vi "main(Test DQMH modules).vi"() -> ()   [LabVIEW 2018, in "Application.lvlib"] (continued)
        n4329 = Or(x=w9739, y=w9737) -> (x .or. y?=w9738:bool)
        n4330 = case shown="False" w9738 {
          tunnel: [w9767 _] -> w9749
          tunnel: w9746 -> [w9766 _]
          frame False {
            w9755 = T9 {"command"="", "data"=variant} ("element")
            w9754 = "MEAS.mux6_1"
            n4331 = To Variant(anything=T2."mux6_1_channel3_3" ("mux6_1(3wires)_encode")) -> (Variant=w9764:variant)
            n4332 = To Variant(anything=T2."mux6_1_channel3_2" ("mux6_1(3wires)_encode")) -> (Variant=w9762:variant)
            n4333 = Bundle By Name(cluster=w9755, "command"=w9754, "data"=w9762) -> (w9761:T9)
            n4334 = Bundle By Name(cluster=w9755, "command"=w9754, "data"=w9764) -> (w9760:T9)
            n4335 = Bundle By Name(cluster=w9755, "command"="MEAS.DMM dual read") -> (w9758:T9)
            n4336 = Build Array(w9761, w9760, w9758) -> (w9756:T9[])
            n4337 = Reverse 1D Array(array=w9756) -> (reversed array=w9757:T9[])
            n4338 = for {
              tunnel: [w9773] -> w9767 mode=indexing
              tunnel: w9766 -> [w9772]
              tunnel: w9757 -> [w9771] mode=indexing
              n4339 = Unbundle By Name(w9771) -> ("command"=w9770:string, "data"=w9769:variant)
              n4340 = call "App enquece.vi"("Priority Enquece"=TRUE, "command data"=w9769, "command"=w9770, "queue in"=w9772) -> ("error out"=w9773:errorcluster)  [unwired: 6 in, 1 out]
            }
          }
          frame True {
          }
        }
        n4341 = Merge Errors(w9747, w9749) -> (w9748:errorcluster)
      }
      frame "Test DRV 58" {
        w9782 = 58  # DUT index(1-60)
        n4342 = disable-structure shown="LOGGING==TRUE" {
          disable-tunnel: w9783 -> [w9816 _]
          frame condition #0 (active) {
            n4343 = Empty String/Path?(string/path=w9816) -> (empty?=w9818:bool)
            n4344 = Select(t="Quece timeout", s=w9818, f=w9816) -> (s? t:f=w9815:string)
            n4345 = call "string log (SubVI).vi"("state Name"=w9815) -> ()  [unwired: 9 in, 2 out]
          }
          frame condition #1 {
          }
        }
        n4346 = call "progress string(SubVI).vi"("String 3"=w9783, "String in"=w9784) -> ("String out"=w9785:string)  [unwired: 9 in]
        n4347 = call "FGV DRV stand.vi"() -> ("Sub-Test.DCV"=w9781:bool)  [unwired: 10 in, 1 out]
        n4348 = call "FGV Driver Data.vi"("DUT index(1-60)"=w9782) -> ("DUT SC"=w9780:bool)  [unwired: 7 in, 3 out]
        n4349 = Not(x=w9781) -> (.not. x?=w9778:bool)
        n4350 = Or(x=w9780, y=w9778) -> (x .or. y?=w9779:bool)
        n4351 = case shown="False" w9779 {
          tunnel: [w9808 _] -> w9790
          tunnel: w9787 -> [w9807 _]
          frame False {
            w9796 = T9 {"command"="", "data"=variant} ("element")
            w9795 = "MEAS.mux6_1"
            n4352 = To Variant(anything=T2."mux6_1_channel4_3" ("mux6_1(3wires)_encode")) -> (Variant=w9805:variant)
            n4353 = To Variant(anything=T2."mux6_1_channel4_2" ("mux6_1(3wires)_encode")) -> (Variant=w9803:variant)
            n4354 = Bundle By Name(cluster=w9796, "command"=w9795, "data"=w9803) -> (w9802:T9)
            n4355 = Bundle By Name(cluster=w9796, "command"=w9795, "data"=w9805) -> (w9801:T9)
            n4356 = Bundle By Name(cluster=w9796, "command"="MEAS.DMM dual read") -> (w9799:T9)
            n4357 = Build Array(w9802, w9801, w9799) -> (w9797:T9[])
            n4358 = Reverse 1D Array(array=w9797) -> (reversed array=w9798:T9[])
            n4359 = for {
              tunnel: [w9814] -> w9808 mode=indexing
              tunnel: w9807 -> [w9813]
              tunnel: w9798 -> [w9812] mode=indexing
              n4360 = Unbundle By Name(w9812) -> ("command"=w9811:string, "data"=w9810:variant)
              n4361 = call "App enquece.vi"("Priority Enquece"=TRUE, "command data"=w9810, "command"=w9811, "queue in"=w9813) -> ("error out"=w9814:errorcluster)  [unwired: 6 in, 1 out]
            }
          }
          frame True {
          }
        }
        n4362 = Merge Errors(w9788, w9790) -> (w9789:errorcluster)
      }
      frame "Test DRV 59" {
        w9823 = 59  # DUT index(1-60)
        n4363 = disable-structure shown="LOGGING==TRUE" {
          disable-tunnel: w9824 -> [w9857 _]
          frame condition #0 (active) {
            n4364 = Empty String/Path?(string/path=w9857) -> (empty?=w9859:bool)
            n4365 = Select(t="Quece timeout", s=w9859, f=w9857) -> (s? t:f=w9856:string)
            n4366 = call "string log (SubVI).vi"("state Name"=w9856) -> ()  [unwired: 9 in, 2 out]
          }
          frame condition #1 {
          }
        }
        n4367 = call "progress string(SubVI).vi"("String 3"=w9824, "String in"=w9825) -> ("String out"=w9826:string)  [unwired: 9 in]
        n4368 = call "FGV DRV stand.vi"() -> ("Sub-Test.DCV"=w9822:bool)  [unwired: 10 in, 1 out]
        n4369 = call "FGV Driver Data.vi"("DUT index(1-60)"=w9823) -> ("DUT SC"=w9821:bool)  [unwired: 7 in, 3 out]
        n4370 = Not(x=w9822) -> (.not. x?=w9819:bool)
        n4371 = Or(x=w9821, y=w9819) -> (x .or. y?=w9820:bool)
        n4372 = case shown="False" w9820 {
          tunnel: [w9849 _] -> w9831
          tunnel: w9828 -> [w9848 _]
          frame False {
            w9837 = T9 {"command"="", "data"=variant} ("element")
            w9836 = "MEAS.mux6_1"
            n4373 = To Variant(anything=T2."mux6_1_channel5_3" ("mux6_1(3wires)_encode")) -> (Variant=w9846:variant)
            n4374 = To Variant(anything=T2."mux6_1_channel5_2" ("mux6_1(3wires)_encode")) -> (Variant=w9844:variant)
            n4375 = Bundle By Name(cluster=w9837, "command"=w9836, "data"=w9844) -> (w9843:T9)
            n4376 = Bundle By Name(cluster=w9837, "command"=w9836, "data"=w9846) -> (w9842:T9)
            n4377 = Bundle By Name(cluster=w9837, "command"="MEAS.DMM dual read") -> (w9840:T9)
            n4378 = Build Array(w9843, w9842, w9840) -> (w9838:T9[])
            n4379 = Reverse 1D Array(array=w9838) -> (reversed array=w9839:T9[])
            n4380 = for {
              tunnel: [w9855] -> w9849 mode=indexing
              tunnel: w9848 -> [w9854]
              tunnel: w9839 -> [w9853] mode=indexing
              n4381 = Unbundle By Name(w9853) -> ("command"=w9852:string, "data"=w9851:variant)
              n4382 = call "App enquece.vi"("Priority Enquece"=TRUE, "command data"=w9851, "command"=w9852, "queue in"=w9854) -> ("error out"=w9855:errorcluster)  [unwired: 6 in, 1 out]
            }
          }
          frame True {
          }
        }
        n4383 = Merge Errors(w9829, w9831) -> (w9830:errorcluster)
      }
      frame "Test DRV 60" {
        w9864 = 60  # DUT index(1-60)
        n4384 = disable-structure shown="LOGGING==TRUE" {
          disable-tunnel: w9865 -> [w9898 _]
          frame condition #0 (active) {
            n4385 = Empty String/Path?(string/path=w9898) -> (empty?=w9900:bool)
            n4386 = Select(t="Quece timeout", s=w9900, f=w9898) -> (s? t:f=w9897:string)
            n4387 = call "string log (SubVI).vi"("state Name"=w9897) -> ()  [unwired: 9 in, 2 out]
          }
          frame condition #1 {
          }
        }
        n4388 = call "progress string(SubVI).vi"("String 3"=w9865, "String in"=w9866) -> ("String out"=w9867:string)  [unwired: 9 in]
        n4389 = call "FGV DRV stand.vi"() -> ("Sub-Test.DCV"=w9863:bool)  [unwired: 10 in, 1 out]
        n4390 = call "FGV Driver Data.vi"("DUT index(1-60)"=w9864) -> ("DUT SC"=w9862:bool)  [unwired: 7 in, 3 out]
        n4391 = Not(x=w9863) -> (.not. x?=w9860:bool)
        n4392 = Or(x=w9862, y=w9860) -> (x .or. y?=w9861:bool)
        n4393 = case shown="False" w9861 {
          tunnel: [w9890 _] -> w9872
          tunnel: w9869 -> [w9889 _]
          frame False {
            w9878 = T9 {"command"="", "data"=variant} ("element")
            w9877 = "MEAS.mux6_1"
            n4394 = To Variant(anything=T2."mux6_1_channel6_3" ("mux6_1(3wires)_encode")) -> (Variant=w9887:variant)
            n4395 = To Variant(anything=T2."mux6_1_channel6_2" ("mux6_1(3wires)_encode")) -> (Variant=w9885:variant)
            n4396 = Bundle By Name(cluster=w9878, "command"=w9877, "data"=w9885) -> (w9884:T9)
            n4397 = Bundle By Name(cluster=w9878, "command"=w9877, "data"=w9887) -> (w9883:T9)
            n4398 = Bundle By Name(cluster=w9878, "command"="MEAS.DMM dual read") -> (w9881:T9)
            n4399 = Build Array(w9884, w9883, w9881) -> (w9879:T9[])
            n4400 = Reverse 1D Array(array=w9879) -> (reversed array=w9880:T9[])
            n4401 = for {
              tunnel: [w9896] -> w9890 mode=indexing
              tunnel: w9889 -> [w9895]
              tunnel: w9880 -> [w9894] mode=indexing
              n4402 = Unbundle By Name(w9894) -> ("command"=w9893:string, "data"=w9892:variant)
              n4403 = call "App enquece.vi"("Priority Enquece"=TRUE, "command data"=w9892, "command"=w9893, "queue in"=w9895) -> ("error out"=w9896:errorcluster)  [unwired: 6 in, 1 out]
            }
          }
          frame True {
          }
        }
        n4404 = Merge Errors(w9870, w9872) -> (w9871:errorcluster)
      }
      frame "separated" {
      }
      frame "Test DRV 1A" {
        w9911 = 1 ("DUT index(0-59)")
        n4405 = disable-structure shown="LOGGING==TRUE" {
          disable-tunnel: w9916 -> [w9999 _]
          frame condition #0 (active) {
            n4406 = Empty String/Path?(string/path=w9999) -> (empty?=w10001:bool)
            n4407 = Select(t="Quece timeout", s=w10001, f=w9999) -> (s? t:f=w9998:string)
            n4408 = call "string log (SubVI).vi"("state Name"=w9998) -> ()  [unwired: 9 in, 2 out]
          }
          frame condition #1 {
          }
        }
        n4409 = Flush Queue(queue=w9917) -> (queue out=w9918:refnum<queue>)  [unwired: 1 in, 2 out]
        n4410 = Decrement(x=w9911) -> (x-1=w9915:i32)
        n4411 = Index Array(array=w9912, index=w9915) -> (element=w9913:refnum<vi>)
        n4412 = call "FGV Driver Data.vi"("DUT index(1-60)"=w9911) -> ("DUT SC"=w9909:bool)  [unwired: 7 in, 3 out]
        n4413 = property class="ColBox"(reference=w9913, "Value"=u32 10000536 ("DRV 1")) -> ()  [unwired: 1 in, 2 out]
        n4414 = case shown="False" w9909 {
          tunnel: w9911 -> [w9929 _]
          tunnel: [w9928 w9994] -> w9910
          frame False {
            n4415 = call "FGV DRV stand.vi"() -> ("Sub-Test.DCV"=w9927:bool)  [unwired: 10 in, 1 out]
            n4416 = case shown="False" w9927 {
              tunnel: w9929 -> [w9947 w9966]
              tunnel: [w9946 w9965] -> w9928
              frame False {
                w9930 = T9 {"command"="", "data"=variant} ("element")
                w9945 = T9 {"command"="", "data"=variant} ("element")
                n4417 = To Variant(anything=T3."mux10_1_channel1" ("mux10_1(x6)_encode")) -> (Variant=w9943:variant)
                n4418 = To Variant(anything=T4."demux1_10_channel1" ("demux1_10(x6)_encode")) -> (Variant=w9939:variant)
                n4419 = To Variant(anything=bool[] [TRUE, FALSE, FALSE, FALSE, FALSE, FALSE]) -> (Variant=w9955:variant)
                n4420 = Bundle By Name(cluster=w9945, "command"="MEAS.AllRelaysOFF") -> (w9954:T9)
                n4421 = Bundle By Name(cluster=w9945, "command"="MEAS.mux10-1", "data"=w9943) -> (w9936:T9)
                n4422 = Bundle By Name(cluster=w9945, "command"="MEAS.demux1-10", "data"=w9939) -> (w9937:T9)
                n4423 = Bundle By Name(cluster=w9945, "command"="MEAS.eMIC", "data"=w9955) -> (w9938:T9)
                n4424 = Build Array(w9954, w9936, w9937, w9938) -> (w9932:T9[])
                n4425 = To Variant(anything=w9947) -> (Variant=w9935:variant)
                n4426 = To Variant(anything=w9947) -> (Variant=w9934:variant)
                n4427 = Bundle By Name(cluster=w9930, "command"="WaitFor") -> (w9931:T9)
                n4428 = Bundle By Name(cluster=w9930, "command"="MEAS.requestAC", "data"=w9935) -> (w9952:T9)
                n4429 = Bundle By Name(cluster=w9930, "command"="Apps.WaitForEvent", "data"=w9934) -> (w9948:T9)
                n4430 = Bundle By Name(cluster=w9930, "command"="Apps.UI Update 1") -> (w9949:T9)
                n4431 = Build Array (concatenate)(w9932, w9931, w9952, w9948, w9949) -> (w9946:T9[])
              }
              frame True {
                w9962 = T9 {"command"="", "data"=variant} ("element")
                w9984 = T9 {"command"="", "data"=variant} ("element")
                n4432 = To Variant(anything=T3."mux10_1_channel1" ("mux10_1(x6)_encode")) -> (Variant=w9991:variant)
                n4433 = To Variant(anything=T2."mux6_1_channel1_3" ("mux6_1(3wires)_encode")) -> (Variant=w9989:variant)
                n4434 = To Variant(anything=T4."demux1_10_channel1" ("demux1_10(x6)_encode")) -> (Variant=w9985:variant)
                n4435 = To Variant(anything=bool[] [TRUE, FALSE, FALSE, FALSE, FALSE, FALSE]) -> (Variant=w9981:variant)
                n4436 = Bundle By Name(cluster=w9984, "command"="MEAS.AllRelaysOFF") -> (w9980:T9)
                n4437 = Bundle By Name(cluster=w9984, "command"="MEAS.mux10-1", "data"=w9991) -> (w9979:T9)
                n4438 = Bundle By Name(cluster=w9984, "command"="MEAS.mux6_1", "data"=w9989) -> (w9978:T9)
                n4439 = Bundle By Name(cluster=w9984, "command"="MEAS.demux1-10", "data"=w9985) -> (w9977:T9)
                n4440 = Bundle By Name(cluster=w9984, "command"="MEAS.eMIC", "data"=w9981) -> (w9976:T9)
                n4441 = Build Array(w9980, w9979, w9978, w9977, w9976) -> (w9960:T9[])
                n4442 = To Variant(anything=w9966) -> (Variant=w9964:variant)
                n4443 = To Variant(anything=w9966) -> (Variant=w9963:variant)
                n4444 = Bundle By Name(cluster=w9962, "command"="WaitFor") -> (w9959:T9)
                n4445 = Bundle By Name(cluster=w9962, "command"="MEAS.DMM dual read") -> (w9973:T9)
                n4446 = Bundle By Name(cluster=w9962, "command"="MEAS.requestAC", "data"=w9964) -> (w9972:T9)
                n4447 = Bundle By Name(cluster=w9962, "command"="Apps.WaitForEvent", "data"=w9963) -> (w9967:T9)
                n4448 = Bundle By Name(cluster=w9962, "command"="Apps.UI Update 1") -> (w9968:T9)
                n4449 = Build Array (concatenate)(w9960, w9959, w9973, w9972, w9967, w9968) -> (w9965:T9[])
              }
            }
          }
          frame True {
            n4450 = Bundle By Name(cluster=T9 {"command"="", "data"=variant} ("element"), "command"="Apps.UI Update 1") -> (w9995:T9)
            n4451 = Build Array(w9995) -> (w9994:T9[])
          }
        }
        n4452 = for {
          tunnel: w9910 -> [w10005] mode=indexing
          tunnel: w9918 -> [w10006]
          tunnel: [w10002] -> w9920 mode=indexing
          n4453 = Unbundle By Name(w10005) -> ("command"=w10004:string, "data"=w10003:variant)
          n4454 = call "App enquece.vi"("command data"=w10003, "command"=w10004, "queue in"=w10006) -> ("error out"=w10002:errorcluster)  [unwired: 7 in, 1 out]
        }
        n4455 = Merge Errors(w9921, w9920) -> (w9919:errorcluster)
      }
      frame "Test DRV 2A" {
        w10009 = 2 ("DUT index(0-59)")
        n4456 = disable-structure shown="LOGGING==TRUE" {
          disable-tunnel: w10014 -> [w10097 _]
          frame condition #0 (active) {
            n4457 = Empty String/Path?(string/path=w10097) -> (empty?=w10099:bool)
            n4458 = Select(t="Quece timeout", s=w10099, f=w10097) -> (s? t:f=w10096:string)
            n4459 = call "string log (SubVI).vi"("state Name"=w10096) -> ()  [unwired: 9 in, 2 out]
          }
          frame condition #1 {
          }
        }
        n4460 = Flush Queue(queue=w10015) -> (queue out=w10016:refnum<queue>)  [unwired: 1 in, 2 out]
        n4461 = Decrement(x=w10009) -> (x-1=w10013:i32)
        n4462 = Index Array(array=w10010, index=w10013) -> (element=w10011:refnum<vi>)
        n4463 = property class="ColBox"(reference=w10011, "Value"=u32 10000536 ("DRV 1")) -> ()  [unwired: 1 in, 2 out]
        n4464 = call "FGV Driver Data.vi"("DUT index(1-60)"=w10009) -> ("DUT SC"=w10007:bool)  [unwired: 7 in, 3 out]
        n4465 = case shown="False" w10007 {
          tunnel: w10009 -> [w10027 _]
          tunnel: [w10026 w10092] -> w10008
          frame False {
            n4466 = call "FGV DRV stand.vi"() -> ("Sub-Test.DCV"=w10025:bool)  [unwired: 10 in, 1 out]
            n4467 = case shown="True" w10025 {
              tunnel: w10027 -> [w10045 w10064]
              tunnel: [w10044 w10063] -> w10026
              frame False {
                w10031 = T9 {"command"="", "data"=variant} ("element")
                w10043 = T9 {"command"="", "data"=variant} ("element")
                n4468 = To Variant(anything=T3."mux10_1_channel1" ("mux10_1(x6)_encode")) -> (Variant=w10041:variant)
                n4469 = To Variant(anything=T4."demux1_10_channel1" ("demux1_10(x6)_encode")) -> (Variant=w10037:variant)
                n4470 = To Variant(anything=bool[] [FALSE, TRUE, FALSE, FALSE, FALSE, FALSE]) -> (Variant=w10053:variant)
                n4471 = Bundle By Name(cluster=w10043, "command"="MEAS.AllRelaysOFF") -> (w10052:T9)
                n4472 = Bundle By Name(cluster=w10043, "command"="MEAS.mux10-1", "data"=w10041) -> (w10034:T9)
                n4473 = Bundle By Name(cluster=w10043, "command"="MEAS.demux1-10", "data"=w10037) -> (w10035:T9)
                n4474 = Bundle By Name(cluster=w10043, "command"="MEAS.eMIC", "data"=w10053) -> (w10036:T9)
                n4475 = Build Array(w10052, w10034, w10035, w10036) -> (w10030:T9[])
                n4476 = To Variant(anything=w10045) -> (Variant=w10033:variant)
                n4477 = To Variant(anything=w10045) -> (Variant=w10032:variant)
                n4478 = Bundle By Name(cluster=w10031, "command"="WaitFor") -> (w10029:T9)
                n4479 = Bundle By Name(cluster=w10031, "command"="MEAS.requestAC", "data"=w10033) -> (w10050:T9)
                n4480 = Bundle By Name(cluster=w10031, "command"="Apps.WaitForEvent", "data"=w10032) -> (w10046:T9)
                n4481 = Bundle By Name(cluster=w10031, "command"="Apps.UI Update 1") -> (w10047:T9)
                n4482 = Build Array (concatenate)(w10030, w10029, w10050, w10046, w10047) -> (w10044:T9[])
              }
              frame True {
                w10060 = T9 {"command"="", "data"=variant} ("element")
                w10082 = T9 {"command"="", "data"=variant} ("element")
                n4483 = To Variant(anything=T3."mux10_1_channel1" ("mux10_1(x6)_encode")) -> (Variant=w10089:variant)
                n4484 = To Variant(anything=T2."mux6_1_channel2_3" ("mux6_1(3wires)_encode")) -> (Variant=w10087:variant)
                n4485 = To Variant(anything=T4."demux1_10_channel1" ("demux1_10(x6)_encode")) -> (Variant=w10083:variant)
                n4486 = To Variant(anything=bool[] [FALSE, TRUE, FALSE, FALSE, FALSE, FALSE]) -> (Variant=w10079:variant)
                n4487 = Bundle By Name(cluster=w10082, "command"="MEAS.AllRelaysOFF") -> (w10078:T9)
                n4488 = Bundle By Name(cluster=w10082, "command"="MEAS.mux10-1", "data"=w10089) -> (w10077:T9)
                n4489 = Bundle By Name(cluster=w10082, "command"="MEAS.mux6_1", "data"=w10087) -> (w10076:T9)
                n4490 = Bundle By Name(cluster=w10082, "command"="MEAS.demux1-10", "data"=w10083) -> (w10075:T9)
                n4491 = Bundle By Name(cluster=w10082, "command"="MEAS.eMIC", "data"=w10079) -> (w10074:T9)
                n4492 = Build Array(w10078, w10077, w10076, w10075, w10074) -> (w10058:T9[])
                n4493 = To Variant(anything=w10064) -> (Variant=w10062:variant)
                n4494 = To Variant(anything=w10064) -> (Variant=w10061:variant)
                n4495 = Bundle By Name(cluster=w10060, "command"="WaitFor") -> (w10057:T9)
                n4496 = Bundle By Name(cluster=w10060, "command"="MEAS.DMM dual read") -> (w10071:T9)
                n4497 = Bundle By Name(cluster=w10060, "command"="MEAS.requestAC", "data"=w10062) -> (w10070:T9)
                n4498 = Bundle By Name(cluster=w10060, "command"="Apps.WaitForEvent", "data"=w10061) -> (w10065:T9)
                n4499 = Bundle By Name(cluster=w10060, "command"="Apps.UI Update 1") -> (w10066:T9)
                n4500 = Build Array (concatenate)(w10058, w10057, w10071, w10070, w10065, w10066) -> (w10063:T9[])
              }
            }
          }
          frame True {
            n4501 = Bundle By Name(cluster=T9 {"command"="", "data"=variant} ("element"), "command"="Apps.UI Update 1") -> (w10093:T9)
            n4502 = Build Array(w10093) -> (w10092:T9[])
          }
        }
        n4503 = for {
          tunnel: w10008 -> [w10103] mode=indexing
          tunnel: w10016 -> [w10104]
          tunnel: [w10100] -> w10018 mode=indexing
          n4504 = Unbundle By Name(w10103) -> ("command"=w10102:string, "data"=w10101:variant)
          n4505 = call "App enquece.vi"("command data"=w10101, "command"=w10102, "queue in"=w10104) -> ("error out"=w10100:errorcluster)  [unwired: 7 in, 1 out]
        }
        n4506 = Merge Errors(w10019, w10018) -> (w10017:errorcluster)
      }
      frame "Test DRV 3A" {
        w10107 = 3 ("DUT index(0-59)")
        n4507 = disable-structure shown="LOGGING==TRUE" {
          disable-tunnel: w10112 -> [w10195 _]
          frame condition #0 (active) {
            n4508 = Empty String/Path?(string/path=w10195) -> (empty?=w10197:bool)
            n4509 = Select(t="Quece timeout", s=w10197, f=w10195) -> (s? t:f=w10194:string)
            n4510 = call "string log (SubVI).vi"("state Name"=w10194) -> ()  [unwired: 9 in, 2 out]
          }
          frame condition #1 {
          }
        }
        n4511 = Flush Queue(queue=w10113) -> (queue out=w10114:refnum<queue>)  [unwired: 1 in, 2 out]
        n4512 = Decrement(x=w10107) -> (x-1=w10111:i32)
        n4513 = Index Array(array=w10108, index=w10111) -> (element=w10109:refnum<vi>)
        n4514 = property class="ColBox"(reference=w10109, "Value"=u32 10000536 ("DRV 1")) -> ()  [unwired: 1 in, 2 out]
        n4515 = call "FGV Driver Data.vi"("DUT index(1-60)"=w10107) -> ("DUT SC"=w10105:bool)  [unwired: 7 in, 3 out]
        n4516 = case shown="False" w10105 {
          tunnel: w10107 -> [w10125 _]
          tunnel: [w10124 w10190] -> w10106
          frame False {
            n4517 = call "FGV DRV stand.vi"() -> ("Sub-Test.DCV"=w10123:bool)  [unwired: 10 in, 1 out]
            n4518 = case shown="True" w10123 {
              tunnel: w10125 -> [w10143 w10162]
              tunnel: [w10142 w10161] -> w10124
              frame False {
                w10128 = T9 {"command"="", "data"=variant} ("element")
                w10141 = T9 {"command"="", "data"=variant} ("element")
                n4519 = To Variant(anything=T3."mux10_1_channel1" ("mux10_1(x6)_encode")) -> (Variant=w10139:variant)
                n4520 = To Variant(anything=T4."demux1_10_channel1" ("demux1_10(x6)_encode")) -> (Variant=w10135:variant)
                n4521 = To Variant(anything=bool[] [FALSE, FALSE, TRUE, FALSE, FALSE, FALSE]) -> (Variant=w10151:variant)
                n4522 = Bundle By Name(cluster=w10141, "command"="MEAS.AllRelaysOFF") -> (w10150:T9)
                n4523 = Bundle By Name(cluster=w10141, "command"="MEAS.mux10-1", "data"=w10139) -> (w10132:T9)
                n4524 = Bundle By Name(cluster=w10141, "command"="MEAS.demux1-10", "data"=w10135) -> (w10133:T9)
                n4525 = Bundle By Name(cluster=w10141, "command"="MEAS.eMIC", "data"=w10151) -> (w10134:T9)
                n4526 = Build Array(w10150, w10132, w10133, w10134) -> (w10127:T9[])
                n4527 = To Variant(anything=w10143) -> (Variant=w10131:variant)
                n4528 = To Variant(anything=w10143) -> (Variant=w10130:variant)
                n4529 = Bundle By Name(cluster=w10128, "command"="WaitFor") -> (w10126:T9)
                n4530 = Bundle By Name(cluster=w10128, "command"="MEAS.requestAC", "data"=w10131) -> (w10148:T9)
                n4531 = Bundle By Name(cluster=w10128, "command"="Apps.WaitForEvent", "data"=w10130) -> (w10144:T9)
                n4532 = Bundle By Name(cluster=w10128, "command"="Apps.UI Update 1") -> (w10145:T9)
                n4533 = Build Array (concatenate)(w10127, w10126, w10148, w10144, w10145) -> (w10142:T9[])
              }
              frame True {
                w10158 = T9 {"command"="", "data"=variant} ("element")
                w10180 = T9 {"command"="", "data"=variant} ("element")
                n4534 = To Variant(anything=T3."mux10_1_channel1" ("mux10_1(x6)_encode")) -> (Variant=w10187:variant)
                n4535 = To Variant(anything=T2."mux6_1_channel3_3" ("mux6_1(3wires)_encode")) -> (Variant=w10185:variant)
                n4536 = To Variant(anything=T4."demux1_10_channel1" ("demux1_10(x6)_encode")) -> (Variant=w10181:variant)
                n4537 = To Variant(anything=bool[] [FALSE, FALSE, TRUE, FALSE, FALSE, FALSE]) -> (Variant=w10177:variant)
                n4538 = Bundle By Name(cluster=w10180, "command"="MEAS.AllRelaysOFF") -> (w10176:T9)
                n4539 = Bundle By Name(cluster=w10180, "command"="MEAS.mux10-1", "data"=w10187) -> (w10175:T9)
                n4540 = Bundle By Name(cluster=w10180, "command"="MEAS.mux6_1", "data"=w10185) -> (w10174:T9)
                n4541 = Bundle By Name(cluster=w10180, "command"="MEAS.demux1-10", "data"=w10181) -> (w10173:T9)
                n4542 = Bundle By Name(cluster=w10180, "command"="MEAS.eMIC", "data"=w10177) -> (w10172:T9)
                n4543 = Build Array(w10176, w10175, w10174, w10173, w10172) -> (w10156:T9[])
                n4544 = To Variant(anything=w10162) -> (Variant=w10160:variant)
                n4545 = To Variant(anything=w10162) -> (Variant=w10159:variant)
                n4546 = Bundle By Name(cluster=w10158, "command"="WaitFor") -> (w10155:T9)
                n4547 = Bundle By Name(cluster=w10158, "command"="MEAS.DMM dual read") -> (w10169:T9)
                n4548 = Bundle By Name(cluster=w10158, "command"="MEAS.requestAC", "data"=w10160) -> (w10168:T9)
                n4549 = Bundle By Name(cluster=w10158, "command"="Apps.WaitForEvent", "data"=w10159) -> (w10163:T9)
                n4550 = Bundle By Name(cluster=w10158, "command"="Apps.UI Update 1") -> (w10164:T9)
                n4551 = Build Array (concatenate)(w10156, w10155, w10169, w10168, w10163, w10164) -> (w10161:T9[])
              }
            }
          }
          frame True {
            n4552 = Bundle By Name(cluster=T9 {"command"="", "data"=variant} ("element"), "command"="Apps.UI Update 1") -> (w10191:T9)
            n4553 = Build Array(w10191) -> (w10190:T9[])
          }
        }
        n4554 = for {
          tunnel: w10106 -> [w10201] mode=indexing
          tunnel: w10114 -> [w10202]
          tunnel: [w10198] -> w10116 mode=indexing
          n4555 = Unbundle By Name(w10201) -> ("command"=w10200:string, "data"=w10199:variant)
          n4556 = call "App enquece.vi"("command data"=w10199, "command"=w10200, "queue in"=w10202) -> ("error out"=w10198:errorcluster)  [unwired: 7 in, 1 out]
        }
        n4557 = Merge Errors(w10117, w10116) -> (w10115:errorcluster)
      }
      frame "Test DRV 4A" {
        w10207 = 4 ("DUT index(0-59)")
        n4558 = disable-structure shown="LOGGING==TRUE" {
          disable-tunnel: w10210 -> [w10293 _]
          frame condition #0 (active) {
            n4559 = Empty String/Path?(string/path=w10293) -> (empty?=w10295:bool)
            n4560 = Select(t="Quece timeout", s=w10295, f=w10293) -> (s? t:f=w10292:string)
            n4561 = call "string log (SubVI).vi"("state Name"=w10292) -> ()  [unwired: 9 in, 2 out]
          }
          frame condition #1 {
          }
        }
        n4562 = Flush Queue(queue=w10211) -> (queue out=w10212:refnum<queue>)  [unwired: 1 in, 2 out]
        n4563 = Decrement(x=w10207) -> (x-1=w10209:i32)
        n4564 = Index Array(array=w10208, index=w10209) -> (element=w10204:refnum<vi>)
        n4565 = call "FGV Driver Data.vi"("DUT index(1-60)"=w10207) -> ("DUT SC"=w10205:bool)  [unwired: 7 in, 3 out]
        n4566 = property class="ColBox"(reference=w10204, "Value"=u32 10000536 ("DRV 1")) -> ()  [unwired: 1 in, 2 out]
        n4567 = case shown="False" w10205 {
          tunnel: w10207 -> [w10223 _]
          tunnel: [w10222 w10288] -> w10206
          frame False {
            n4568 = call "FGV DRV stand.vi"() -> ("Sub-Test.DCV"=w10221:bool)  [unwired: 10 in, 1 out]
            n4569 = case shown="True" w10221 {
              tunnel: w10223 -> [w10241 w10260]
              tunnel: [w10240 w10259] -> w10222
              frame False {
                w10224 = T9 {"command"="", "data"=variant} ("element")
                w10239 = T9 {"command"="", "data"=variant} ("element")
                n4570 = To Variant(anything=T3."mux10_1_channel1" ("mux10_1(x6)_encode")) -> (Variant=w10237:variant)
                n4571 = To Variant(anything=T4."demux1_10_channel1" ("demux1_10(x6)_encode")) -> (Variant=w10233:variant)
                n4572 = To Variant(anything=bool[] [FALSE, FALSE, FALSE, TRUE, FALSE, FALSE]) -> (Variant=w10249:variant)
                n4573 = Bundle By Name(cluster=w10239, "command"="MEAS.AllRelaysOFF") -> (w10248:T9)
                n4574 = Bundle By Name(cluster=w10239, "command"="MEAS.mux10-1", "data"=w10237) -> (w10230:T9)
                n4575 = Bundle By Name(cluster=w10239, "command"="MEAS.demux1-10", "data"=w10233) -> (w10231:T9)
                n4576 = Bundle By Name(cluster=w10239, "command"="MEAS.eMIC", "data"=w10249) -> (w10232:T9)
                n4577 = Build Array(w10248, w10230, w10231, w10232) -> (w10226:T9[])
                n4578 = To Variant(anything=w10241) -> (Variant=w10229:variant)
                n4579 = To Variant(anything=w10241) -> (Variant=w10228:variant)
                n4580 = Bundle By Name(cluster=w10224, "command"="WaitFor") -> (w10225:T9)
                n4581 = Bundle By Name(cluster=w10224, "command"="MEAS.requestAC", "data"=w10229) -> (w10246:T9)
                n4582 = Bundle By Name(cluster=w10224, "command"="Apps.WaitForEvent", "data"=w10228) -> (w10242:T9)
                n4583 = Bundle By Name(cluster=w10224, "command"="Apps.UI Update 1") -> (w10243:T9)
                n4584 = Build Array (concatenate)(w10226, w10225, w10246, w10242, w10243) -> (w10240:T9[])
              }
              frame True {
                w10255 = T9 {"command"="", "data"=variant} ("element")
                w10278 = T9 {"command"="", "data"=variant} ("element")
                n4585 = To Variant(anything=T3."mux10_1_channel1" ("mux10_1(x6)_encode")) -> (Variant=w10285:variant)
                n4586 = To Variant(anything=T2."mux6_1_channel4_3" ("mux6_1(3wires)_encode")) -> (Variant=w10283:variant)
                n4587 = To Variant(anything=T4."demux1_10_channel1" ("demux1_10(x6)_encode")) -> (Variant=w10279:variant)
                n4588 = To Variant(anything=bool[] [FALSE, FALSE, FALSE, TRUE, FALSE, FALSE]) -> (Variant=w10275:variant)
                n4589 = Bundle By Name(cluster=w10278, "command"="MEAS.AllRelaysOFF") -> (w10274:T9)
                n4590 = Bundle By Name(cluster=w10278, "command"="MEAS.mux10-1", "data"=w10285) -> (w10273:T9)
                n4591 = Bundle By Name(cluster=w10278, "command"="MEAS.mux6_1", "data"=w10283) -> (w10272:T9)
                n4592 = Bundle By Name(cluster=w10278, "command"="MEAS.demux1-10", "data"=w10279) -> (w10271:T9)
                n4593 = Bundle By Name(cluster=w10278, "command"="MEAS.eMIC", "data"=w10275) -> (w10270:T9)
                n4594 = Build Array(w10274, w10273, w10272, w10271, w10270) -> (w10254:T9[])
                n4595 = To Variant(anything=w10260) -> (Variant=w10258:variant)
                n4596 = To Variant(anything=w10260) -> (Variant=w10257:variant)
                n4597 = Bundle By Name(cluster=w10255, "command"="WaitFor") -> (w10253:T9)
                n4598 = Bundle By Name(cluster=w10255, "command"="MEAS.DMM dual read") -> (w10267:T9)
                n4599 = Bundle By Name(cluster=w10255, "command"="MEAS.requestAC", "data"=w10258) -> (w10266:T9)
                n4600 = Bundle By Name(cluster=w10255, "command"="Apps.WaitForEvent", "data"=w10257) -> (w10261:T9)
                n4601 = Bundle By Name(cluster=w10255, "command"="Apps.UI Update 1") -> (w10262:T9)
                n4602 = Build Array (concatenate)(w10254, w10253, w10267, w10266, w10261, w10262) -> (w10259:T9[])
              }
            }
          }
          frame True {
            n4603 = Bundle By Name(cluster=T9 {"command"="", "data"=variant} ("element"), "command"="Apps.UI Update 1") -> (w10289:T9)
            n4604 = Build Array(w10289) -> (w10288:T9[])
          }
        }
        n4605 = for {
          tunnel: w10206 -> [w10299] mode=indexing
          tunnel: w10212 -> [w10300]
          tunnel: [w10296] -> w10214 mode=indexing
          n4606 = Unbundle By Name(w10299) -> ("command"=w10298:string, "data"=w10297:variant)
          n4607 = call "App enquece.vi"("command data"=w10297, "command"=w10298, "queue in"=w10300) -> ("error out"=w10296:errorcluster)  [unwired: 7 in, 1 out]
        }
        n4608 = Merge Errors(w10215, w10214) -> (w10213:errorcluster)
      }
      frame "Test DRV 5A" {
        w10304 = 5 ("DUT index(0-59)")
        n4609 = disable-structure shown="LOGGING==TRUE" {
          disable-tunnel: w10309 -> [w10392 _]
          frame condition #0 (active) {
            n4610 = Empty String/Path?(string/path=w10392) -> (empty?=w10394:bool)
            n4611 = Select(t="Quece timeout", s=w10394, f=w10392) -> (s? t:f=w10391:string)
            n4612 = call "string log (SubVI).vi"("state Name"=w10391) -> ()  [unwired: 9 in, 2 out]
          }
          frame condition #1 {
          }
        }
        n4613 = Flush Queue(queue=w10310) -> (queue out=w10311:refnum<queue>)  [unwired: 1 in, 2 out]
        n4614 = Decrement(x=w10304) -> (x-1=w10308:i32)
        n4615 = Index Array(array=w10305, index=w10308) -> (element=w10306:refnum<vi>)
        n4616 = call "FGV DRV stand.vi"() -> ("Sub-Test.DCV"=w10301:bool)  [unwired: 10 in, 1 out]
        n4617 = call "FGV Driver Data.vi"("DUT index(1-60)"=w10304) -> ("DUT SC"=w10302:bool)  [unwired: 7 in, 3 out]
        n4618 = property class="ColBox"(reference=w10306, "Value"=u32 10000536 ("DRV 1")) -> ()  [unwired: 1 in, 2 out]
        n4619 = case shown="False" w10302 {
          tunnel: w10304 -> [w10322 _]
          tunnel: [w10321 w10387] -> w10303
          tunnel: w10301 -> [w10320 _]
          frame False {
            n4620 = case shown="False" w10320 {
              tunnel: w10322 -> [w10329 w10359]
              tunnel: [w10340 w10358] -> w10321
              frame False {
                w10326 = T9 {"command"="", "data"=variant} ("element")
                w10339 = T9 {"command"="", "data"=variant} ("element")
                n4621 = To Variant(anything=T3."mux10_1_channel1" ("mux10_1(x6)_encode")) -> (Variant=w10337:variant)
                n4622 = To Variant(anything=T4."demux1_10_channel1" ("demux1_10(x6)_encode")) -> (Variant=w10333:variant)
                n4623 = To Variant(anything=bool[] [FALSE, FALSE, FALSE, FALSE, TRUE, FALSE]) -> (Variant=w10348:variant)
                n4624 = Bundle By Name(cluster=w10339, "command"="MEAS.AllRelaysOFF") -> (w10347:T9)
                n4625 = Bundle By Name(cluster=w10339, "command"="MEAS.mux10-1", "data"=w10337) -> (w10330:T9)
                n4626 = Bundle By Name(cluster=w10339, "command"="MEAS.demux1-10", "data"=w10333) -> (w10331:T9)
                n4627 = Bundle By Name(cluster=w10339, "command"="MEAS.eMIC", "data"=w10348) -> (w10332:T9)
                n4628 = Build Array(w10347, w10330, w10331, w10332) -> (w10325:T9[])
                n4629 = To Variant(anything=w10329) -> (Variant=w10328:variant)
                n4630 = To Variant(anything=w10329) -> (Variant=w10327:variant)
                n4631 = Bundle By Name(cluster=w10326, "command"="MEAS.requestAC", "data"=w10328) -> (w10345:T9)
                n4632 = Bundle By Name(cluster=w10326, "command"="Apps.WaitForEvent", "data"=w10327) -> (w10341:T9)
                n4633 = Bundle By Name(cluster=w10326, "command"="Apps.UI Update 1") -> (w10342:T9)
                n4634 = Bundle By Name(cluster=w10326, "command"="WaitFor") -> (w10324:T9)
                n4635 = Build Array (concatenate)(w10325, w10324, w10345, w10341, w10342) -> (w10340:T9[])
              }
              frame True {
                w10355 = T9 {"command"="", "data"=variant} ("element")
                w10377 = T9 {"command"="", "data"=variant} ("element")
                n4636 = To Variant(anything=T3."mux10_1_channel1" ("mux10_1(x6)_encode")) -> (Variant=w10384:variant)
                n4637 = To Variant(anything=T2."mux6_1_channel5_3" ("mux6_1(3wires)_encode")) -> (Variant=w10382:variant)
                n4638 = To Variant(anything=T4."demux1_10_channel1" ("demux1_10(x6)_encode")) -> (Variant=w10378:variant)
                n4639 = To Variant(anything=bool[] [FALSE, FALSE, FALSE, FALSE, TRUE, FALSE]) -> (Variant=w10374:variant)
                n4640 = Bundle By Name(cluster=w10377, "command"="MEAS.AllRelaysOFF") -> (w10373:T9)
                n4641 = Bundle By Name(cluster=w10377, "command"="MEAS.mux10-1", "data"=w10384) -> (w10372:T9)
                n4642 = Bundle By Name(cluster=w10377, "command"="MEAS.mux6_1", "data"=w10382) -> (w10371:T9)
                n4643 = Bundle By Name(cluster=w10377, "command"="MEAS.demux1-10", "data"=w10378) -> (w10370:T9)
                n4644 = Bundle By Name(cluster=w10377, "command"="MEAS.eMIC", "data"=w10374) -> (w10369:T9)
                n4645 = Build Array(w10373, w10372, w10371, w10370, w10369) -> (w10354:T9[])
                n4646 = To Variant(anything=w10359) -> (Variant=w10357:variant)
                n4647 = To Variant(anything=w10359) -> (Variant=w10356:variant)
                n4648 = Bundle By Name(cluster=w10355, "command"="WaitFor") -> (w10353:T9)
                n4649 = Bundle By Name(cluster=w10355, "command"="MEAS.DMM dual read") -> (w10366:T9)
                n4650 = Bundle By Name(cluster=w10355, "command"="MEAS.requestAC", "data"=w10357) -> (w10365:T9)
                n4651 = Bundle By Name(cluster=w10355, "command"="Apps.WaitForEvent", "data"=w10356) -> (w10360:T9)
                n4652 = Bundle By Name(cluster=w10355, "command"="Apps.UI Update 1") -> (w10361:T9)
                n4653 = Build Array (concatenate)(w10354, w10353, w10366, w10365, w10360, w10361) -> (w10358:T9[])
              }
            }
          }
          frame True {
            n4654 = Bundle By Name(cluster=T9 {"command"="", "data"=variant} ("element"), "command"="Apps.UI Update 1") -> (w10388:T9)
            n4655 = Build Array(w10388) -> (w10387:T9[])
          }
        }
        n4656 = for {
          tunnel: w10303 -> [w10398] mode=indexing
          tunnel: w10311 -> [w10399]
          tunnel: [w10395] -> w10313 mode=indexing
          n4657 = Unbundle By Name(w10398) -> ("command"=w10397:string, "data"=w10396:variant)
          n4658 = call "App enquece.vi"("command data"=w10396, "command"=w10397, "queue in"=w10399) -> ("error out"=w10395:errorcluster)  [unwired: 7 in, 1 out]
        }
        n4659 = Merge Errors(w10314, w10313) -> (w10312:errorcluster)
      }
      frame "Test DRV 6A" {
        w10403 = 6 ("DUT index(0-59)")
        n4660 = disable-structure shown="LOGGING==TRUE" {
          disable-tunnel: w10408 -> [w10491 _]
          frame condition #0 (active) {
            n4661 = Empty String/Path?(string/path=w10491) -> (empty?=w10493:bool)
            n4662 = Select(t="Quece timeout", s=w10493, f=w10491) -> (s? t:f=w10490:string)
            n4663 = call "string log (SubVI).vi"("state Name"=w10490) -> ()  [unwired: 9 in, 2 out]
          }
          frame condition #1 {
          }
        }
        n4664 = Flush Queue(queue=w10409) -> (queue out=w10410:refnum<queue>)  [unwired: 1 in, 2 out]
        n4665 = Decrement(x=w10403) -> (x-1=w10407:i32)
        n4666 = Index Array(array=w10404, index=w10407) -> (element=w10405:refnum<vi>)
        n4667 = call "FGV DRV stand.vi"() -> ("Sub-Test.DCV"=w10400:bool)  [unwired: 10 in, 1 out]
        n4668 = call "FGV Driver Data.vi"("DUT index(1-60)"=w10403) -> ("DUT SC"=w10401:bool)  [unwired: 7 in, 3 out]
        n4669 = property class="ColBox"(reference=w10405, "Value"=u32 10000536 ("DRV 1")) -> ()  [unwired: 1 in, 2 out]
        n4670 = case shown="False" w10401 {
          tunnel: w10403 -> [w10421 _]
          tunnel: [w10420 w10486] -> w10402
          tunnel: w10400 -> [w10419 _]
          frame False {
            n4671 = case shown="True" w10419 {
              tunnel: w10421 -> [w10428 w10458]
              tunnel: [w10439 w10457] -> w10420
              frame False {
                w10425 = T9 {"command"="", "data"=variant} ("element")
                w10438 = T9 {"command"="", "data"=variant} ("element")
                n4672 = To Variant(anything=T3."mux10_1_channel1" ("mux10_1(x6)_encode")) -> (Variant=w10436:variant)
                n4673 = To Variant(anything=T4."demux1_10_channel1" ("demux1_10(x6)_encode")) -> (Variant=w10432:variant)
                n4674 = To Variant(anything=bool[] [FALSE, FALSE, FALSE, FALSE, FALSE, TRUE]) -> (Variant=w10447:variant)
                n4675 = Bundle By Name(cluster=w10438, "command"="MEAS.AllRelaysOFF") -> (w10446:T9)
                n4676 = Bundle By Name(cluster=w10438, "command"="MEAS.mux10-1", "data"=w10436) -> (w10429:T9)
                n4677 = Bundle By Name(cluster=w10438, "command"="MEAS.demux1-10", "data"=w10432) -> (w10430:T9)
                n4678 = Bundle By Name(cluster=w10438, "command"="MEAS.eMIC", "data"=w10447) -> (w10431:T9)
                n4679 = Build Array(w10446, w10429, w10430, w10431) -> (w10424:T9[])
                n4680 = To Variant(anything=w10428) -> (Variant=w10427:variant)
                n4681 = To Variant(anything=w10428) -> (Variant=w10426:variant)
                n4682 = Bundle By Name(cluster=w10425, "command"="MEAS.requestAC", "data"=w10427) -> (w10444:T9)
                n4683 = Bundle By Name(cluster=w10425, "command"="Apps.WaitForEvent", "data"=w10426) -> (w10440:T9)
                n4684 = Bundle By Name(cluster=w10425, "command"="Apps.UI Update 1") -> (w10441:T9)
                n4685 = Bundle By Name(cluster=w10425, "command"="WaitFor") -> (w10423:T9)
                n4686 = Build Array (concatenate)(w10424, w10423, w10444, w10440, w10441) -> (w10439:T9[])
              }
              frame True {
                w10454 = T9 {"command"="", "data"=variant} ("element")
                w10476 = T9 {"command"="", "data"=variant} ("element")
                n4687 = To Variant(anything=T3."mux10_1_channel1" ("mux10_1(x6)_encode")) -> (Variant=w10483:variant)
                n4688 = To Variant(anything=T2."mux6_1_channel6_3" ("mux6_1(3wires)_encode")) -> (Variant=w10481:variant)
                n4689 = To Variant(anything=T4."demux1_10_channel1" ("demux1_10(x6)_encode")) -> (Variant=w10477:variant)
                n4690 = To Variant(anything=bool[] [FALSE, FALSE, FALSE, FALSE, FALSE, TRUE]) -> (Variant=w10473:variant)
                n4691 = Bundle By Name(cluster=w10476, "command"="MEAS.AllRelaysOFF") -> (w10472:T9)
                n4692 = Bundle By Name(cluster=w10476, "command"="MEAS.mux10-1", "data"=w10483) -> (w10471:T9)
                n4693 = Bundle By Name(cluster=w10476, "command"="MEAS.mux6_1", "data"=w10481) -> (w10470:T9)
                n4694 = Bundle By Name(cluster=w10476, "command"="MEAS.demux1-10", "data"=w10477) -> (w10469:T9)
                n4695 = Bundle By Name(cluster=w10476, "command"="MEAS.eMIC", "data"=w10473) -> (w10468:T9)
                n4696 = Build Array(w10472, w10471, w10470, w10469, w10468) -> (w10453:T9[])
                n4697 = To Variant(anything=w10458) -> (Variant=w10456:variant)
                n4698 = To Variant(anything=w10458) -> (Variant=w10455:variant)
                n4699 = Bundle By Name(cluster=w10454, "command"="WaitFor") -> (w10452:T9)
                n4700 = Bundle By Name(cluster=w10454, "command"="MEAS.DMM dual read") -> (w10465:T9)
                n4701 = Bundle By Name(cluster=w10454, "command"="MEAS.requestAC", "data"=w10456) -> (w10464:T9)
                n4702 = Bundle By Name(cluster=w10454, "command"="Apps.WaitForEvent", "data"=w10455) -> (w10459:T9)
                n4703 = Bundle By Name(cluster=w10454, "command"="Apps.UI Update 1") -> (w10460:T9)
                n4704 = Build Array (concatenate)(w10453, w10452, w10465, w10464, w10459, w10460) -> (w10457:T9[])
              }
            }
          }
          frame True {
            n4705 = Bundle By Name(cluster=T9 {"command"="", "data"=variant} ("element"), "command"="Apps.UI Update 1") -> (w10487:T9)
            n4706 = Build Array(w10487) -> (w10486:T9[])
          }
        }
        n4707 = for {
          tunnel: w10402 -> [w10497] mode=indexing
          tunnel: w10410 -> [w10498]
          tunnel: [w10494] -> w10412 mode=indexing
          n4708 = Unbundle By Name(w10497) -> ("command"=w10496:string, "data"=w10495:variant)
          n4709 = call "App enquece.vi"("command data"=w10495, "command"=w10496, "queue in"=w10498) -> ("error out"=w10494:errorcluster)  [unwired: 7 in, 1 out]
        }
        n4710 = Merge Errors(w10413, w10412) -> (w10411:errorcluster)
      }
      frame "Test DRV 7A" {
        w10502 = 7 ("DUT index(0-59)")
        n4711 = disable-structure shown="LOGGING==TRUE" {
          disable-tunnel: w10507 -> [w10590 _]
          frame condition #0 (active) {
            n4712 = Empty String/Path?(string/path=w10590) -> (empty?=w10592:bool)
            n4713 = Select(t="Quece timeout", s=w10592, f=w10590) -> (s? t:f=w10589:string)
            n4714 = call "string log (SubVI).vi"("state Name"=w10589) -> ()  [unwired: 9 in, 2 out]
          }
          frame condition #1 {
          }
        }
        n4715 = Flush Queue(queue=w10508) -> (queue out=w10509:refnum<queue>)  [unwired: 1 in, 2 out]
        n4716 = Decrement(x=w10502) -> (x-1=w10506:i32)
        n4717 = Index Array(array=w10503, index=w10506) -> (element=w10504:refnum<vi>)
        n4718 = call "FGV DRV stand.vi"() -> ("Sub-Test.DCV"=w10499:bool)  [unwired: 10 in, 1 out]
        n4719 = call "FGV Driver Data.vi"("DUT index(1-60)"=w10502) -> ("DUT SC"=w10500:bool)  [unwired: 7 in, 3 out]
        n4720 = property class="ColBox"(reference=w10504, "Value"=u32 10000536 ("DRV 1")) -> ()  [unwired: 1 in, 2 out]
        n4721 = case shown="False" w10500 {
          tunnel: w10502 -> [w10520 _]
          tunnel: [w10519 w10585] -> w10501
          tunnel: w10499 -> [w10518 _]
          frame False {
            n4722 = case shown="True" w10518 {
              tunnel: w10520 -> [w10527 w10557]
              tunnel: [w10538 w10556] -> w10519
              frame False {
                w10524 = T9 {"command"="", "data"=variant} ("element")
                w10537 = T9 {"command"="", "data"=variant} ("element")
                n4723 = To Variant(anything=T3."mux10_1_channel2" ("mux10_1(x6)_encode")) -> (Variant=w10535:variant)
                n4724 = To Variant(anything=T4."demux1_10_channel2" ("demux1_10(x6)_encode")) -> (Variant=w10531:variant)
                n4725 = To Variant(anything=bool[] [TRUE, FALSE, FALSE, FALSE, FALSE, FALSE]) -> (Variant=w10546:variant)
                n4726 = Bundle By Name(cluster=w10537, "command"="MEAS.AllRelaysOFF") -> (w10545:T9)
                n4727 = Bundle By Name(cluster=w10537, "command"="MEAS.mux10-1", "data"=w10535) -> (w10528:T9)
                n4728 = Bundle By Name(cluster=w10537, "command"="MEAS.demux1-10", "data"=w10531) -> (w10529:T9)
                n4729 = Bundle By Name(cluster=w10537, "command"="MEAS.eMIC", "data"=w10546) -> (w10530:T9)
                n4730 = Build Array(w10545, w10528, w10529, w10530) -> (w10523:T9[])
                n4731 = To Variant(anything=w10527) -> (Variant=w10526:variant)
                n4732 = To Variant(anything=w10527) -> (Variant=w10525:variant)
                n4733 = Bundle By Name(cluster=w10524, "command"="MEAS.requestAC", "data"=w10526) -> (w10543:T9)
                n4734 = Bundle By Name(cluster=w10524, "command"="Apps.WaitForEvent", "data"=w10525) -> (w10539:T9)
                n4735 = Bundle By Name(cluster=w10524, "command"="Apps.UI Update 1") -> (w10540:T9)
                n4736 = Bundle By Name(cluster=w10524, "command"="WaitFor") -> (w10522:T9)
                n4737 = Build Array (concatenate)(w10523, w10522, w10543, w10539, w10540) -> (w10538:T9[])
              }
              frame True {
                w10553 = T9 {"command"="", "data"=variant} ("element")
                w10575 = T9 {"command"="", "data"=variant} ("element")
                n4738 = To Variant(anything=T3."mux10_1_channel2" ("mux10_1(x6)_encode")) -> (Variant=w10582:variant)
                n4739 = To Variant(anything=T2."mux6_1_channel1_3" ("mux6_1(3wires)_encode")) -> (Variant=w10580:variant)
                n4740 = To Variant(anything=T4."demux1_10_channel2" ("demux1_10(x6)_encode")) -> (Variant=w10576:variant)
                n4741 = To Variant(anything=bool[] [TRUE, FALSE, FALSE, FALSE, FALSE, FALSE]) -> (Variant=w10572:variant)
                n4742 = Bundle By Name(cluster=w10575, "command"="MEAS.AllRelaysOFF") -> (w10571:T9)
                n4743 = Bundle By Name(cluster=w10575, "command"="MEAS.mux10-1", "data"=w10582) -> (w10570:T9)
                n4744 = Bundle By Name(cluster=w10575, "command"="MEAS.mux6_1", "data"=w10580) -> (w10569:T9)
                n4745 = Bundle By Name(cluster=w10575, "command"="MEAS.demux1-10", "data"=w10576) -> (w10568:T9)
                n4746 = Bundle By Name(cluster=w10575, "command"="MEAS.eMIC", "data"=w10572) -> (w10567:T9)
                n4747 = Build Array(w10571, w10570, w10569, w10568, w10567) -> (w10552:T9[])
                n4748 = To Variant(anything=w10557) -> (Variant=w10555:variant)
                n4749 = To Variant(anything=w10557) -> (Variant=w10554:variant)
                n4750 = Bundle By Name(cluster=w10553, "command"="WaitFor") -> (w10551:T9)
                n4751 = Bundle By Name(cluster=w10553, "command"="MEAS.DMM dual read") -> (w10564:T9)
                n4752 = Bundle By Name(cluster=w10553, "command"="MEAS.requestAC", "data"=w10555) -> (w10563:T9)
                n4753 = Bundle By Name(cluster=w10553, "command"="Apps.WaitForEvent", "data"=w10554) -> (w10558:T9)
                n4754 = Bundle By Name(cluster=w10553, "command"="Apps.UI Update 1") -> (w10559:T9)
                n4755 = Build Array (concatenate)(w10552, w10551, w10564, w10563, w10558, w10559) -> (w10556:T9[])
              }
            }
          }
          frame True {
            n4756 = Bundle By Name(cluster=T9 {"command"="", "data"=variant} ("element"), "command"="Apps.UI Update 1") -> (w10586:T9)
            n4757 = Build Array(w10586) -> (w10585:T9[])
          }
        }
        n4758 = for {
          tunnel: w10501 -> [w10596] mode=indexing
          tunnel: w10509 -> [w10597]
          tunnel: [w10593] -> w10511 mode=indexing
          n4759 = Unbundle By Name(w10596) -> ("command"=w10595:string, "data"=w10594:variant)
          n4760 = call "App enquece.vi"("command data"=w10594, "command"=w10595, "queue in"=w10597) -> ("error out"=w10593:errorcluster)  [unwired: 7 in, 1 out]
        }
        n4761 = Merge Errors(w10512, w10511) -> (w10510:errorcluster)
      }
      frame "Test DRV 8A" {
        w10601 = 8 ("DUT index(0-59)")
        n4762 = disable-structure shown="LOGGING==TRUE" {
          disable-tunnel: w10606 -> [w10689 _]
          frame condition #0 (active) {
            n4763 = Empty String/Path?(string/path=w10689) -> (empty?=w10691:bool)
            n4764 = Select(t="Quece timeout", s=w10691, f=w10689) -> (s? t:f=w10688:string)
            n4765 = call "string log (SubVI).vi"("state Name"=w10688) -> ()  [unwired: 9 in, 2 out]
          }
          frame condition #1 {
          }
        }
        n4766 = Flush Queue(queue=w10607) -> (queue out=w10608:refnum<queue>)  [unwired: 1 in, 2 out]
        n4767 = Decrement(x=w10601) -> (x-1=w10605:i32)
        n4768 = Index Array(array=w10602, index=w10605) -> (element=w10603:refnum<vi>)
        n4769 = call "FGV DRV stand.vi"() -> ("Sub-Test.DCV"=w10598:bool)  [unwired: 10 in, 1 out]
        n4770 = call "FGV Driver Data.vi"("DUT index(1-60)"=w10601) -> ("DUT SC"=w10599:bool)  [unwired: 7 in, 3 out]
        n4771 = property class="ColBox"(reference=w10603, "Value"=u32 10000536 ("DRV 1")) -> ()  [unwired: 1 in, 2 out]
        n4772 = case shown="False" w10599 {
          tunnel: w10601 -> [w10619 _]
          tunnel: [w10618 w10684] -> w10600
          tunnel: w10598 -> [w10617 _]
          frame False {
            n4773 = case shown="False" w10617 {
